vi "main.vi"(3 "Input\nparameters":T2={"Frame rate (ms)"=2000, "Strain name"="N2", "Time t"=0, "State"=enum."Initialize measurement", "Acquisition time"=0.0, "Maximum # images"=100000, "#TTL"=0, "time of third ttl "=100000, "ImSub Value"=0, "Time of last TTL"=0, "# Rows"=2, "# Columns"=2, "number of adjacentTTL"=0, "Sleep Deprivation status"="", "Sleep Detection"=FALSE, "Time of first sleep detection"=0, "# Sleep detections"=0, "Time max # adjacent TTL"=-10000, "Image t-1"=[], "Image t"=[]} {"# Columns" items=["1"=1, "2"=2, "3"=3, "4"=4]; "# Rows" items=["1"=1, "2"=2, "3"=3, "4"=4]}, 5 "Deprivation\nparameters":T5={"Frame Row"=0, "Kstd"=40.0, "# Images for\nsleep detection"=10, "Kmean"=1.5, "Start time of sleep detection (images):"=1000, "Column"=0, "Deprivation \nlength (images)"=3600, "# TTL"=10000, "by x images after first detection"=0, "Between\nTTL pulses"=0, "\nby x detections"=0, "# Total immobility\n detections"=1.0, "After max #\nadjacent TTL"=60, "#TTL SD start\nreference time\n"=0, "Max #\nadjacent TTL"=10000, " Ca2+\nmode"=0} {"Column" items=["1", "2", "3", "4"]; "Frame Row" items=["1", "2", "3", "4"]}) -> ()   [LabVIEW 2011]
uses:
  state.ctl
panel:
  in  "Display\nimage":bool
  out "Intensity Graph 2":u16[][](graph)
  out "Acquisition\nsuccessfull":bool
  in  "Start\nmeasurement":bool
  in  "Frame\nrate":u32=1000
  in  "Trigger mode":u32(ring) items=["Internal", "External"]
  in  "Exposure time (ms)":dbl=5.0 format="%.1f"
  in  "Manual sleep detection":bool
  in  "Shut Down":bool
  in  "First deprivation method":T3={"TTL channel"="Dev1/port2/line6", "Pause time (ms)"=0, "Pulse length (ms)"=15, "# Pulses"=1}
  in  "#TTL change mode":dbl=10000.0
  in  "Second deprivation method":T4={"TTL channel"="Dev1/port2/line7", "Pause time (ms)"=0, "Pulse Length (ms)"=300, "# Pulses"=1}
  in  "Sleep\nRecognition/Control":bool=TRUE
  # "Camera settings"
  # "TTL pulse settings"
  # "Frame rate (ms)"
  # "Sleep deprivation settings"
  # "Control"
  # "Sleep deprivation"
  # "General settings"
  # "Select # of animals"
  # "Row"
  # "Column"
  # "Channel 6 tap magnet"
  # "Channel 7 LED"
  # "Select deprivation animal"
  # "Row"
  # "Column"
  # "Sleep detection parameters"
  # "Sleep deprivation parameters"
  # "Delay deprivation start:"
  # "Pause deprivation (images):"
  # "Stop deprivation after:"
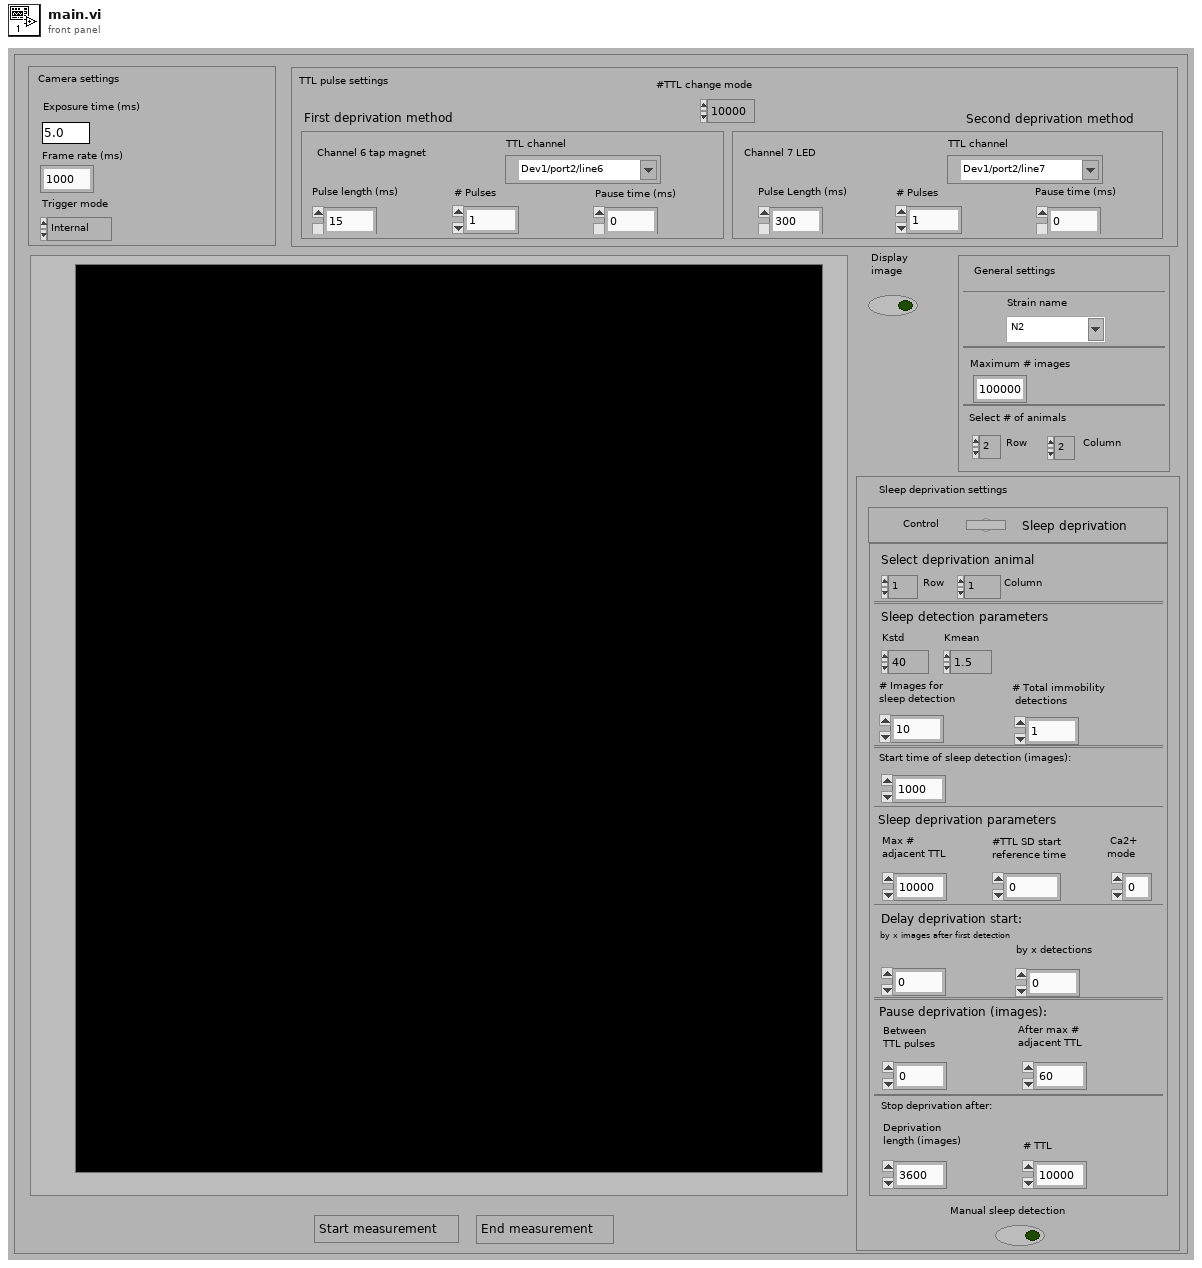
[diagram p1: front panel]
types:
  T1 = typedef "state.ctl" = enum16{"Initialize measurement", "Image acquisition", "Image processing", "Sleep detection", "Control TTL protocol ", "Sleep deprivation", "Update image & exit condition", "Wait "}
  T2 = cluster{"Frame rate (ms)":u32, "Strain name":string, "Time t":i32, "State":T1, "Acquisition time":dbl, "Maximum # images":i32, "#TTL":i32, "time of third ttl ":i32, "ImSub Value":i32, "Time of last TTL":i32, "# Rows":u32, "# Columns":u32, "number of adjacentTTL":i32, "Sleep Deprivation status":string, "Sleep Detection":bool, "Time of first sleep detection":i32, "# Sleep detections":i32, "Time max # adjacent TTL":i32, "Image t-1":i32[][], "Image t":i32[][]}
  T3 = cluster{"TTL channel":tag, "Pause time (ms)":u32, "Pulse length (ms)":u32, "# Pulses":i32}
  T4 = cluster{"TTL channel":tag, "Pause time (ms)":u32, "Pulse Length (ms)":u32, "# Pulses":i32}
  T5 = cluster{"Frame Row":u32, "Kstd":dbl, "# Images for\nsleep detection":i32, "Kmean":dbl, "Start time of sleep detection (images):":i32, "Column":u32, "Deprivation \nlength (images)":i32, "# TTL":i32, "by x images after first detection":i32, "Between\nTTL pulses":i32, "\nby x detections":i32, "# Total immobility\n detections":dbl, "After max #\nadjacent TTL":i32, "#TTL SD start\nreference time\n":i32, "Max #\nadjacent TTL":i32, " Ca2+\nmode":i32}
  T6 = cluster{"Frame rate (ms)":u32, "Worm Strain":string, "Time t":i32, "State":T1, "Acquisition time":dbl, "Maximum # of images":i32, "#TTL":i32, "time of third ttl ":i32, "ImSub Value":i32, "Time of last TTL":i32, "# Rows":u32, "# Columns":u32, "number of adjacentTTL":i32, "Sleep Deprivation status":string, "Sleep Detection":bool, "Time of first sleep detection":i32, "# Sleep detections":i32, "Time max # adjacent TTL":i32, "Image t-1":i32[][], "Image t":i32[][]}
  T7 = cluster{"Frame rate (ms)":u32, "Worm strain":string, "Time t":i32, "State":T1, "Time elapsed":dbl, "Max_num_runs":i32, "#TTL":i32, "Time of start TTL":i32, "ImSub Value":i32, "Time of last TTL":i32, "Number of Columns":u32, "Number of Rows":u32, "# AdjacentTTL":i32, "Sleep deprivation status":string, "Sleep Detection":bool, "# Sleep detections":i32, "Time of first sleep detection":i32, "Time max # adjacent TTL":i32, "Image t-1":i32[][], "Image t":i32[][]}
  T8 = cluster{"Frame rate (ms)":u32, "Worm strain":string, "Time t":i32, "State":T1, "Time elapsed":dbl, "Max_num_runs":i32, "#TTL":i32, "Time of start TTL":i32, "ImSub Value":i32, "Time of last TTL":i32, "Number of Columns":u32, "Number of Rows":u32, "# AdjacentTTL":i32, "Start sleep detection":string, "Sleep Detection":bool, "# Sleep detections":i32, "Time of first sleep detection":i32, "Time max # adjacent TTL":i32, "Image t-1":i32[][], "Image t":i32[][]}
  T9 = cluster{"Frame rate (ms)":u32, "Worm strain":string, "Time t":i32, "State":T1, "Time elapsed":dbl, "Max_num_runs":i32, "#TTL":i32, "Time of start TTL":i32, "ImSub Value":i32, "Time of last TTL":i32, "Number of Columns":u32, "Number of Rows":u32, "# AdjacentTTL":i32, "Sleep deprivation status":string, "Sleep detection":bool, "# Sleep detections":i32, "Time of first sleep detection":i32, "Time max # adjacent TTL":i32, "Image t-1":i32[][], "Image t":i32[][]}
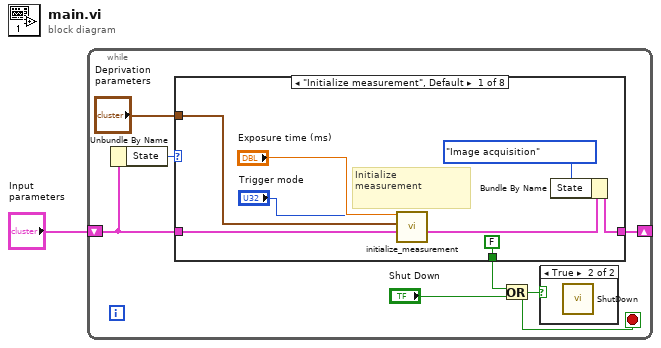
[diagram p0: block diagram]
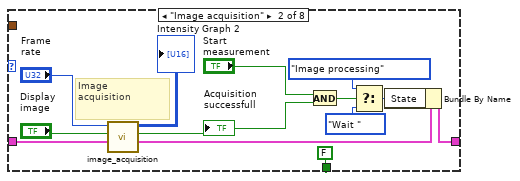
[diagram p3: hidden frame]
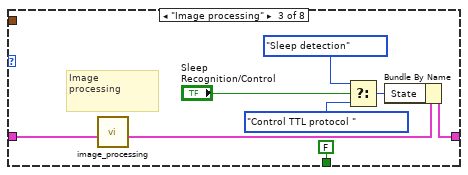
[diagram p4: hidden frame]
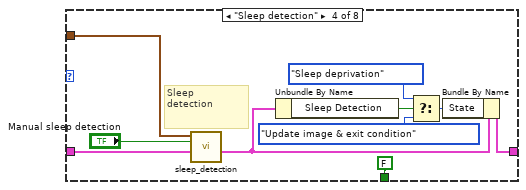
[diagram p5: hidden frame]
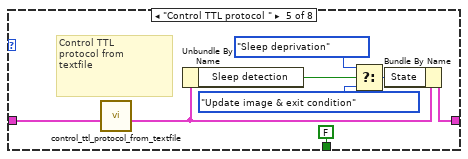
[diagram p6: hidden frame]
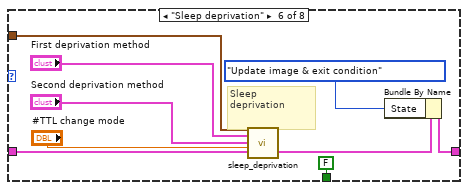
[diagram p7: hidden frame]
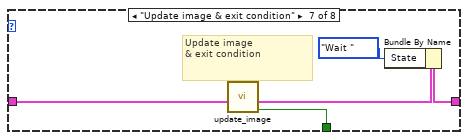
[diagram p8: hidden frame]
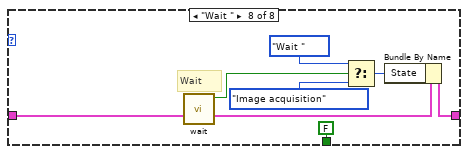
[diagram p9: hidden frame]
diagram:
  n1 = while {
    shift-right: [w8] -> _
    shift-left: "Input\nparameters" -> [w2]
    stop <- w3 stop-if-true
    n2 = Unbundle By Name(w2) -> ("State"=w7:T1)
    n3 = case shown="\"Initialize measurement\", Default" w7 {
      tunnel: [w16 w29 w37 w47 w50 w56 w68 w71] -> w8
      tunnel: w2 -> [w13 w25 w31 w40 w51 w64 w67 w76]
      tunnel: "Deprivation\nparameters" -> [w10 _ _ w41 _ w63 _ _]
      tunnel: [FALSE FALSE FALSE FALSE FALSE FALSE w66 FALSE] -> w4
      frame "Initialize measurement", Default {
        # "Initialize\nmeasurement"
        n4 = call "initialize_measurement.vi"("Trigger\nmode"="Trigger mode", "Deprivation\nsettings"=w10, "Input\nparameters"=w13, "Exposure \ntime"="Exposure time (ms)") -> ("Output\nparameters"=w12:T6)  [unwired: 6 in]
        n5 = Bundle By Name(cluster=w12, "State"=state."Image acquisition") -> (w16:T6)
      }
      frame "Image acquisition" {
        # "Image\nacquisition"
        n6 = call "image_acquisition.vi"("Input\nparameters"=w25, "Display\nImage"="Display\nimage", "Frame\nrate (ms)"="Frame\nrate") -> ("Output\nparameters"=w24:T6, "Acquisition\nsuccessfull"=w19:bool, "Intensity Graph 2"=→"Intensity Graph 2":u16[][])  [unwired: 6 in]
        "Acquisition\nsuccessfull" <- w19
        n7 = And(x="Start\nmeasurement", y=w19) -> (x .and. y?=w20:bool)
        n8 = Select(t=state."Image processing" ("State"), s=w20, f=state."Wait " ("State")) -> (s? t:f=w26:T1)
        n9 = Bundle By Name(cluster=w24, "State"=w26) -> (w29:T6)
      }
      frame "Image processing" {
        # "Image\nprocessing"
        n10 = call "image_processing.vi"("Input\nparameters"=w31) -> ("Output \nparameters"=w30:T7)  [unwired: 10 in]
        n11 = Select(t=state."Sleep detection" ("State"), s="Sleep\nRecognition/Control", f=state."Control TTL protocol " ("State")) -> (s? t:f=w33:T1)
        n12 = Bundle By Name(cluster=w30, "State"=w33) -> (w37:T7)
      }
      frame "Sleep detection" {
        # "Sleep\ndetection"
        n13 = call "sleep_detection.vi"("Deprivation\nparameters"=w41, "Input \nparameters"=w40, "Manual sleep detection"="Manual sleep detection") -> ("Output \nparameters"=w39:T8)  [unwired: 7 in]
        n14 = Unbundle By Name(w39) -> ("Sleep Detection"=w42:bool)
        n15 = Select(t=state."Sleep deprivation" ("State"), s=w42, f=state."Update image & exit condition" ("State")) -> (s? t:f=w43:T1)
        n16 = Bundle By Name(cluster=w39, "State"=w43) -> (w47:T8)
      }
      frame "Control TTL protocol " {
        # "Control TTL\nprotocol from\ntextfile"
        n17 = call "control_ttl_protocol_from_textfile.vi"("Input \nparameters"=w51) -> ("Output \nparameters"=w49:T9)  [unwired: 10 in]
        n18 = Unbundle By Name(w49) -> ("Sleep detection"=w48:bool)
        n19 = Select(t=state."Sleep deprivation" ("State"), s=w48, f=state."Update image & exit condition" ("State")) -> (s? t:f=w52:T1)
        n20 = Bundle By Name(cluster=w49, "State"=w52) -> (w50:T9)
      }
      frame "Sleep deprivation" {
        # "Sleep \ndeprivation"
        n21 = call "sleep_deprivation.vi"("Deprivation\nparameters"=w63, "Input \nparameters"=w64, "#TTL change\nmode"="#TTL change mode", "Second deprivation method"="Second deprivation method", "First deprivation method"="First deprivation method") -> ("Output \nparameters"=w57:T7)  [unwired: 1 in]
        n22 = Bundle By Name(cluster=w57, "State"=state."Update image & exit condition") -> (w56:T7)
      }
      frame "Update image & exit condition" {
        # "Update image\n& exit condition"
        n23 = call "update_image.vi"("Input \nparameters"=w67) -> ("Maximum\ntime reached"=w66:bool, "Output \nparameters"=w65:T7)  [unwired: 9 in]
        n24 = Bundle By Name(cluster=w65, "State"=state."Wait ") -> (w68:T7)
      }
      frame "Wait " {
        # "Wait"
        n25 = call "wait.vi"("Input \nparameters"=w76) -> ("Output \nparameters"=w72:T7, "Wait"=w70:bool)  [unwired: 9 in]
        n26 = Select(t=state."Wait " ("State"), s=w70, f=state."Image acquisition" ("State")) -> (s? t:f=w74:T1)
        n27 = Bundle By Name(cluster=w72, "State"=w74) -> (w71:T7)
      }
    }
    n28 = Or(x=w4, y="Shut Down") -> (x .or. y?=w3:bool)
    n29 = case shown="True" w3 {
      frame False {
      }
      frame True {
        n30 = call <userlib>:"ShutDown.vi"() -> ()  [unwired: 2 in, 2 out]
      }
    }
  }
